vi "CalculateVtopVback.vi"(8 "n_bot":dbl, 11 "n_top":dbl) -> (0 "V_back":dbl, 3 "V_top":dbl)   [LabVIEW 2015]
panel:
  in  "d_eff_top":dbl=3.1
  in  "d_eff_int":dbl=0.85
  in  "d_eff_back":dbl=90.0
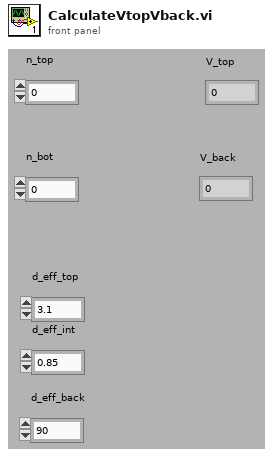
[diagram p1: front panel]
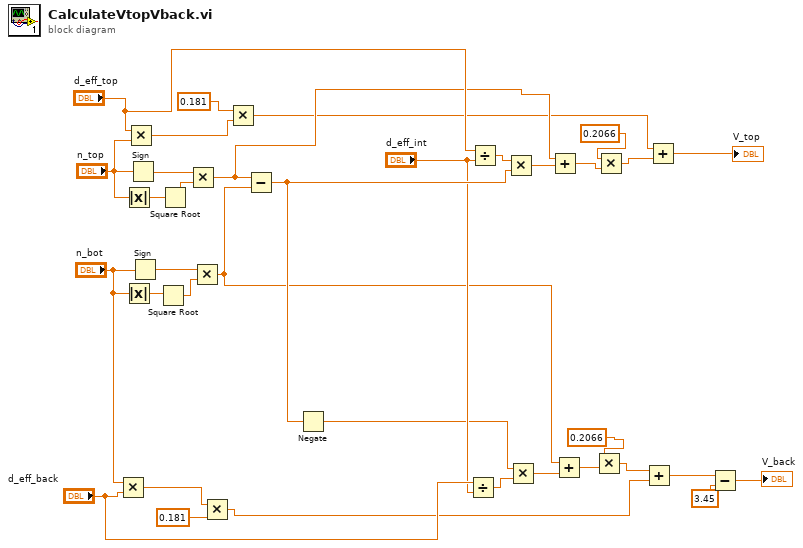
[diagram p0: block diagram]
diagram:
  n1 = Multiply(x="n_bot", y="d_eff_back") -> (x*y=w14:dbl)
  n2 = Absolute Value(x="n_top") -> (abs(x)=w34:dbl)
  n3 = Absolute Value(x="n_bot") -> (abs(x)=w35:dbl)
  n4 = Multiply(x="d_eff_top", y="n_top") -> (x*y=w27:dbl)
  n5 = Sign(1:"n_top") -> (0:w30:dbl)
  n6 = Sign(1:"n_bot") -> (0:w31:dbl)
  n7 = Square Root(x=w35) -> (sqrt(x)=w32:dbl)
  n8 = Square Root(x=w34) -> (sqrt(x)=w33:dbl)
  n9 = Multiply(x=w30, y=w33) -> (x*y=w23:dbl)
  n10 = Multiply(x=w31, y=w32) -> (x*y=w8:dbl)
  n11 = Multiply(x=w14, y=0.181) -> (x*y=w4:dbl)
  n12 = Multiply(x=0.181, y=w27) -> (x*y=w19:dbl)
  n13 = Subtract(x=w23, y=w8) -> (x-y=w17:dbl)
  n14 = Negate(x=w17) -> (-x=w10:dbl)
  n15 = Divide(x="d_eff_back", y="d_eff_int") -> (x/y=w11:dbl)
  n16 = Divide(x="d_eff_top", y="d_eff_int") -> (x/y=w25:dbl)
  n17 = Multiply(x=w25, y=w17) -> (x*y=w24:dbl)
  n18 = Multiply(x=w10, y=w11) -> (x*y=w9:dbl)
  n19 = Add(x=w23, y=w24) -> (x+y=w21:dbl)
  n20 = Add(x=w8, y=w9) -> (x+y=w7:dbl)
  n21 = Multiply(x=0.2066, y=w7) -> (x*y=w5:dbl)
  n22 = Multiply(x=0.2066, y=w21) -> (x*y=w20:dbl)
  n23 = Add(x=w5, y=w4) -> (x+y=w2:dbl)
  n24 = Add(x=w19, y=w20) -> (x+y=→"V_top":dbl)
  n25 = Subtract(x=w2, y=3.45) -> (x-y=→"V_back":dbl)
